vi "Parse URI.vi"(11 "URI":string) -> (0 "path":string, 1 "port":string, 2 "address":string, 3 "protocol":string, 4 "Arguments":cluster{"key":string, "value":string}[](array[cluster]))   [LabVIEW 2014, in "URI.lvlib"]
doc: "JKI State Machine Objects (SMO) 1.3.0.56\nJKI - JKI\nCopyright (c) 2017, JKI"
uses:
  URI.lvlib
  <vilib>/regexp/Match Regular Expression.xnode
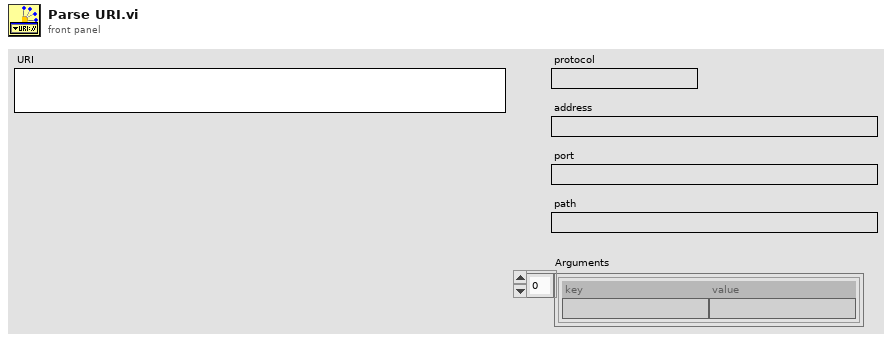
[diagram p1: front panel]
types:
  T1 = cluster{"before match":string, "after match":string}
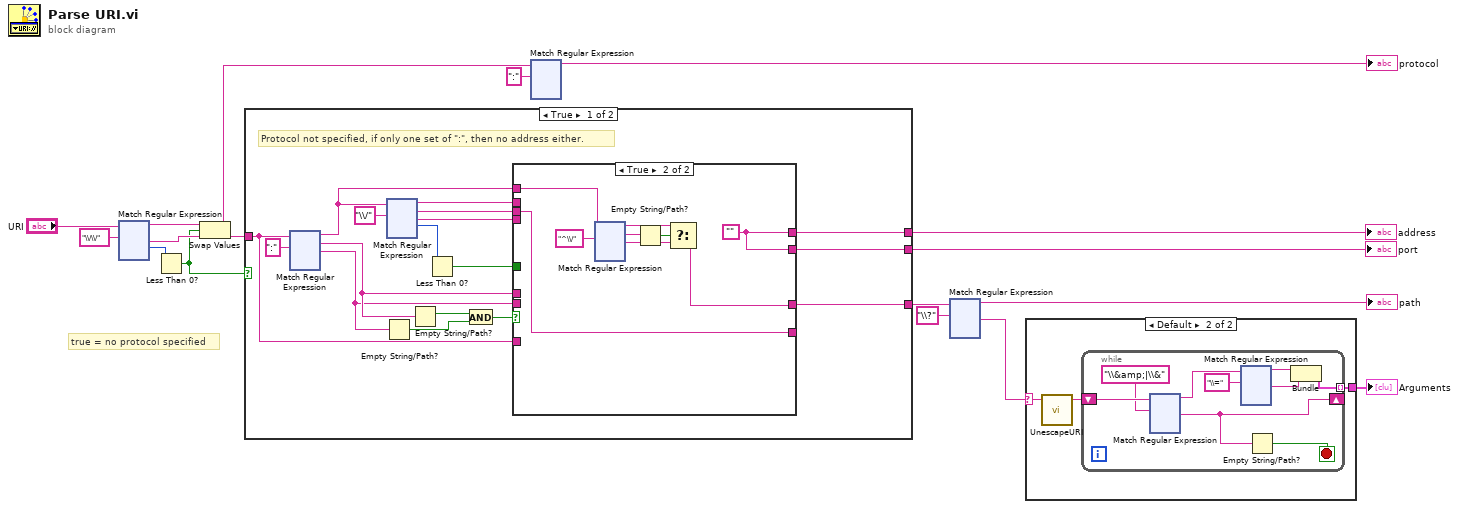
[diagram p0: block diagram]
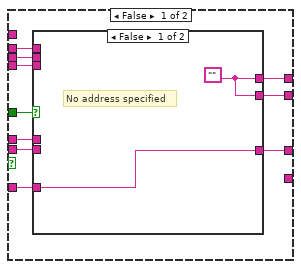
[diagram p3: hidden frame]
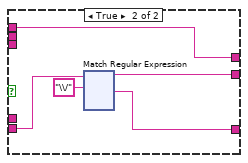
[diagram p4: hidden frame]
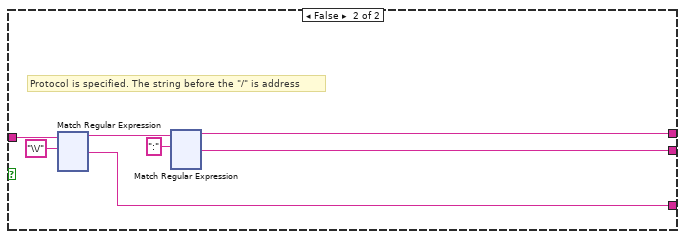
[diagram p5: hidden frame]
diagram:
  # "true = no protocol specified"
  n1 = xnode "Match Regular Expression"("input string"="URI", "regular expression"="\\/\\/") -> ("before match"=w11:string, "after match"=w10:string, "offset past match"=w16:i32)  [unwired: 4 in, 2 out]
  n2 = Less Than 0?(x=w16) -> (x < 0?=w7:bool)
  n3 = Swap Values(12:w11, 13:w7, 14:w10) -> (1:w8:string, 3:w9:string)
  n4 = case shown="True" w7 {
    tunnel: [w27 w522] -> w15
    tunnel: [w26 w520] -> w14
    tunnel: w9 -> [w29 w519]
    tunnel: [w28 w517] -> w3
    frame True {
      # "Protocol not specified, if only one set of \":\", then no address either."
      n5 = xnode "Match Regular Expression"("input string"=w29, "regular expression"=":") -> ("before match"=w18:string, "whole match"=w23:string, "after match"=w22:string)  [unwired: 4 in, 2 out]
      n6 = Empty String/Path?(string/path=w22) -> (empty?=w20:bool)
      n7 = xnode "Match Regular Expression"("input string"=w18, "regular expression"="\\/") -> ("before match"=w30:string, "whole match"=w25:string, "after match"=w31:string, "offset past match"=w32:i32)  [unwired: 4 in, 1 out]
      n8 = Empty String/Path?(string/path=w23) -> (empty?=w21:bool)
      n9 = Less Than 0?(x=w32) -> (x < 0?=w24:bool)
      n10 = And(x=w21, y=w20) -> (x .and. y?=w19:bool)
      n11 = case shown="True" w19 {
        tunnel: w22 -> [w44 _]
        tunnel: w31 -> [w43 _]
        tunnel: w30 -> [w42 _]
        tunnel: w29 -> [w41 _]
        tunnel: [w40 w167] -> w28
        tunnel: [w39 w174] -> w27
        tunnel: [w38 w174] -> w26
        tunnel: w25 -> [w37 w172]
        tunnel: w23 -> [w36 _]
        tunnel: w24 -> [w35 _]
        tunnel: [_ w172] -> _
        tunnel: w18 -> [_ w170]
        frame False {
          n12 = case shown="False" w35 {
            tunnel: w44 -> [_ w49]
            tunnel: w43 -> [_ _]
            tunnel: w42 -> [_ w50]
            tunnel: w41 -> [w46 _]
            tunnel: [w46 w47] -> w40
            tunnel: [w45 w50] -> w39
            tunnel: [w45 w48] -> w38
            tunnel: w36 -> [_ _]
            tunnel: w37 -> [_ _]
            frame False {
              w45 = ""
              # "No address specified"
            }
            frame True {
              n13 = xnode "Match Regular Expression"("input string"=w49, "regular expression"="\\/") -> ("before match"=w48:string, "after match"=w47:string)  [unwired: 4 in, 3 out]
            }
          }
        }
        frame True {
          w174 = ""
          n14 = xnode "Match Regular Expression"("input string"=w170, "regular expression"="^\\/") -> ("before match"=w169:string, "whole match"=w166:string, "after match"=w168:string)  [unwired: 4 in, 2 out]
          n15 = Empty String/Path?(string/path=w166) -> (empty?=w173:bool)
          n16 = Select(t=w169, s=w173, f=w168) -> (s? t:f=w167:string)
        }
      }
    }
    frame False {
      # "Protocol is specified. The string before the \"/\" is address"
      n17 = xnode "Match Regular Expression"("input string"=w519, "regular expression"="\\/") -> ("before match"=w518:string, "after match"=w517:string)  [unwired: 4 in, 3 out]
      n18 = xnode "Match Regular Expression"("input string"=w518, "regular expression"=":") -> ("before match"=w522:string, "after match"=w520:string)  [unwired: 4 in, 3 out]
    }
  }
  "address" <- w15
  "port" <- w14
  n19 = xnode "Match Regular Expression"("input string"=w8, "regular expression"=":") -> ("before match"=→"protocol":string)  [unwired: 4 in, 4 out]
  n20 = xnode "Match Regular Expression"("input string"=w3, "regular expression"="\\?") -> ("before match"=→"path":string, "after match"=w1:string)  [unwired: 4 in, 3 out]
  n21 = case shown="Default" w1 {
    selector: w1 -> [_ w753]
    tunnel: [_ w754] -> w2
    frame "" {
    }
    frame Default {
      n22 = call "UnescapeURI.vi"("Escaped URI"=w753) -> ("URI"=w752:string)  [unwired: 10 in]
      n23 = while {
        tunnel: [w758] -> w754 mode=indexing
        shift-right: [w757] -> _
        shift-left: w752 -> [w763]
        stop <- w756 stop-if-true
        n24 = xnode "Match Regular Expression"("input string"=w763, "regular expression"="\\&amp;|\\&") -> ("before match"=w761:string, "after match"=w757:string)  [unwired: 4 in, 3 out]
        n25 = xnode "Match Regular Expression"("input string"=w761, "regular expression"="\\=") -> ("before match"=w760:string, "after match"=w759:string)  [unwired: 4 in, 3 out]
        n26 = Empty String/Path?(string/path=w757) -> (empty?=w756:bool)
        n27 = Bundle("before match"=w760, "after match"=w759) -> (w758:T1)  [unwired: 1 in]
      }
    }
  }
  "Arguments" <- w2
